vi "Breakdown & Action Taken Report FINAL.vi"(8 "error in (no error)":errorcluster) -> ()   [LabVIEW 2017]
uses:
  <vilib>/Utility/miscctls.llb/LVRowAndColumnTypeDef.ctl
  <vilib>/addons/database/Connection.llb/DB Tools Open Connec (Path).vi
  Globle/Login Details.vi
  <vilib>/Utility/file.llb/Write Delimited Spreadsheet (string).vi
  <vilib>/addons/database/NI_Database_API.lvlib
panel:
  out "Role Id":string
  out "stackholder":string
  in  "Cancel Button - Archive":bool
  out "Table 2":string[][](array[string])
  in  "Manage":bool
  out "Table":string[][](table)
  out "Run-Time Status":cluster{"Array 2":timestamp[], dbl[]}(graph)
  out "index of element":i32
  in  "Download":bool
  in  "Get Rport":bool
  out "subarray":string[](array[string])
  in  "Export to Excel":bool
  in  "Shift":string(combo)
  out "error out":errorcluster
  in  "Station":string(combo)
  in  "To Date":timestamp format="%<%Y-%m-%d>T"
  in  "From Date":timestamp format="%<%Y-%m-%d>T"
  in  "Delete":bool
  in  "Edit":bool
  in  "Select Stakeholder":string(combo)
  in  "Get Report":bool
  # "Breakdown & Action Taken Report"
  # "Designed And Developed By - Infinity Automation Systems Pvt. Ltd."
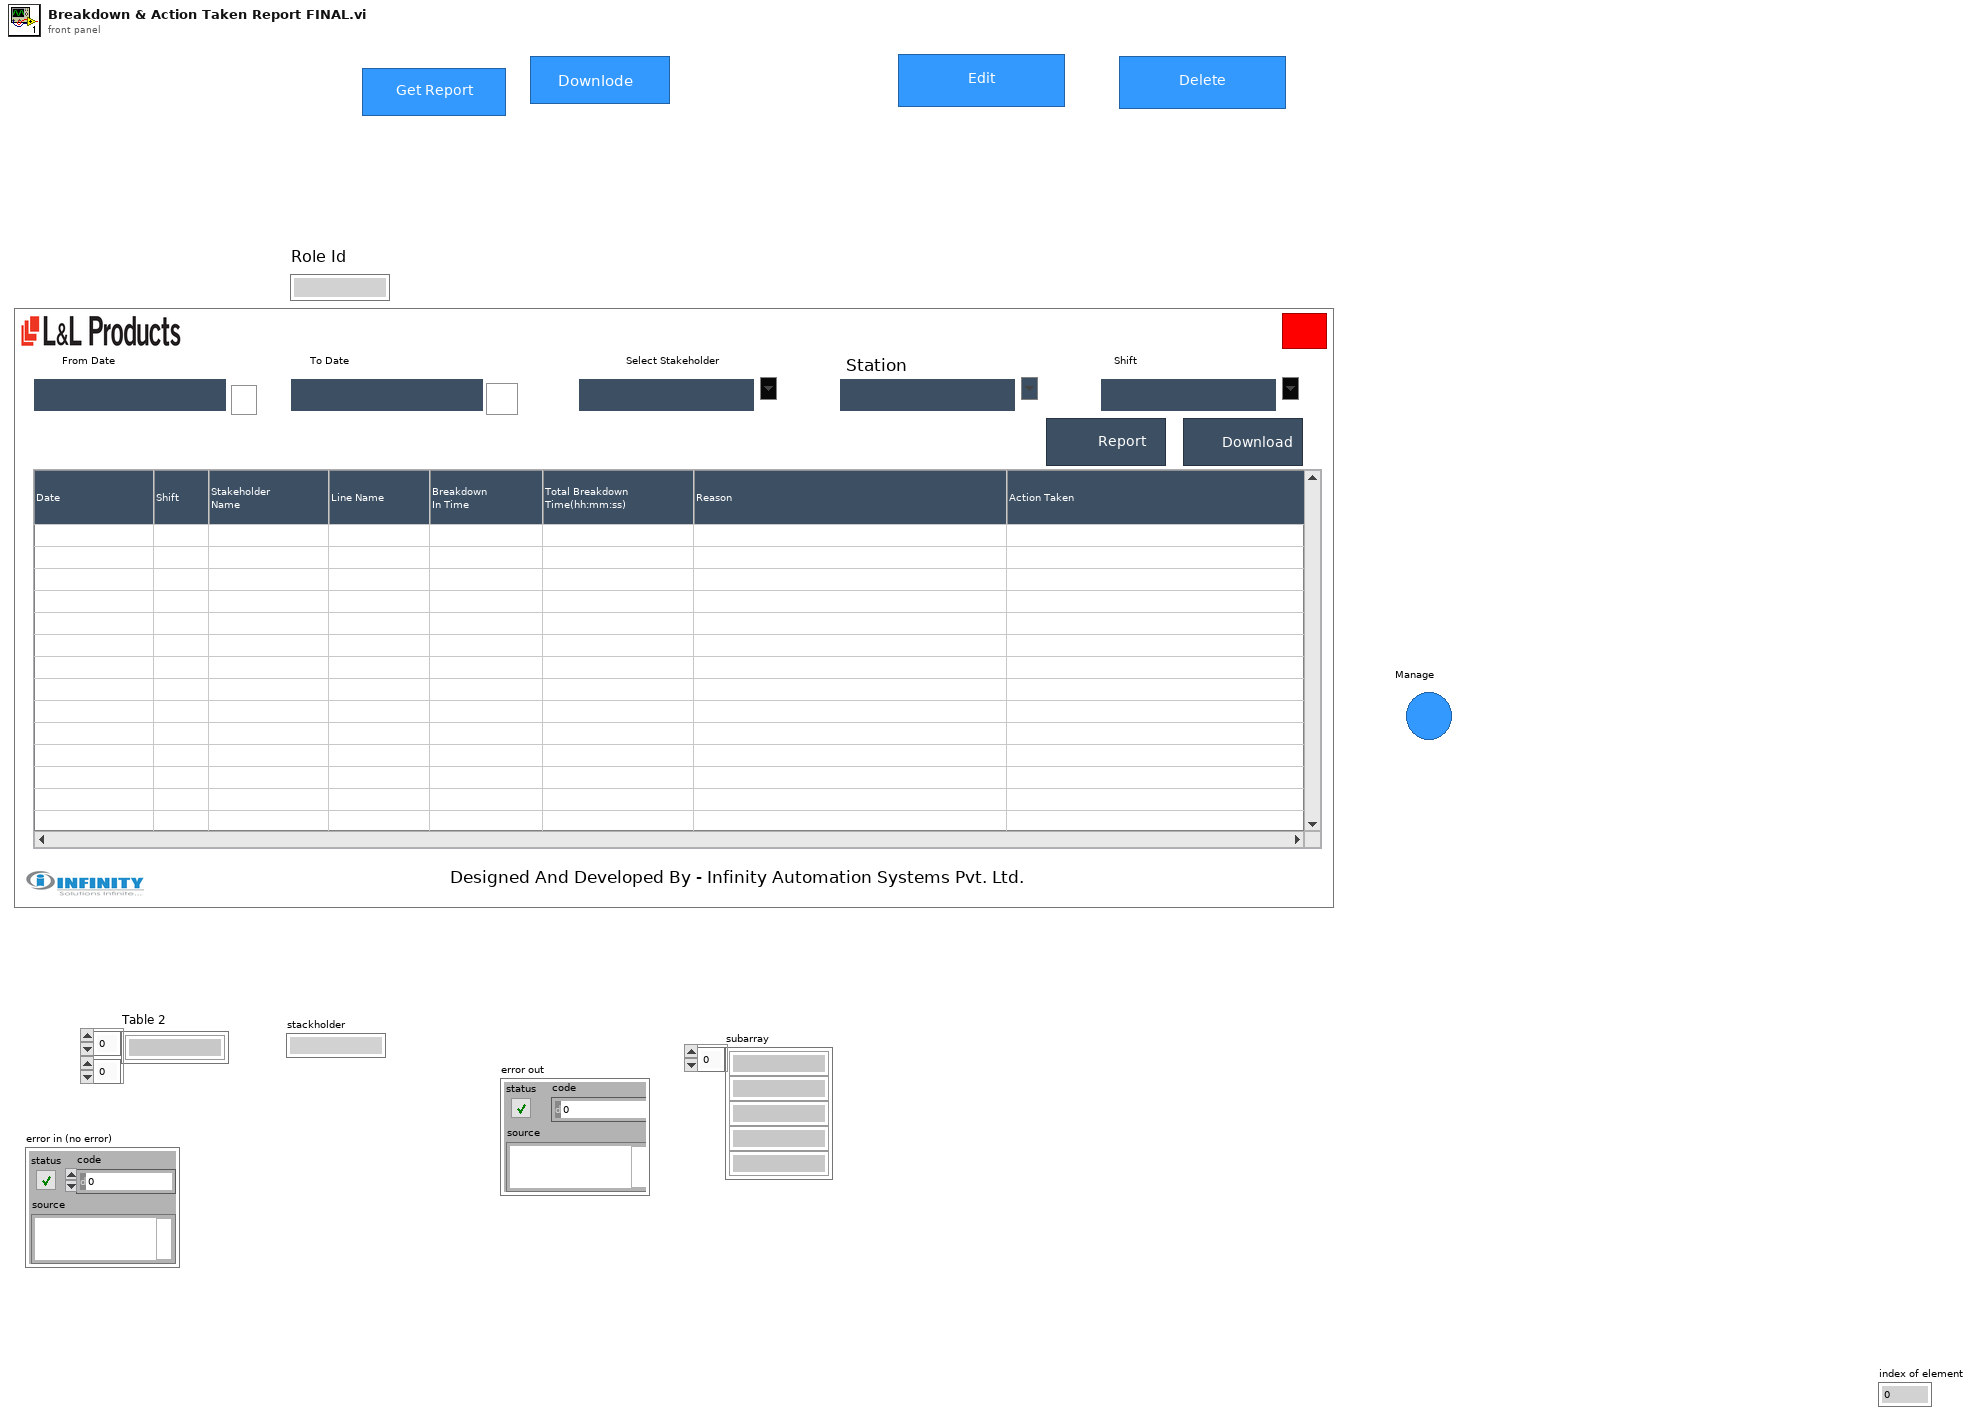
[diagram p1: front panel]
types:
  T1 = typedef "LVRowAndColumnTypeDef.ctl" = cluster{"Row":i32, "Column":i32}
  T2 = typedef "NI_Database_API.lvlib/Conn ObjectReference.ctl" = refnum<k1>
  T3 = enum32{"invalid app kind", "Development System", "Run Time System", "Student Edition", "Embedded LabVIEW", "Evaluation", "Custom"}
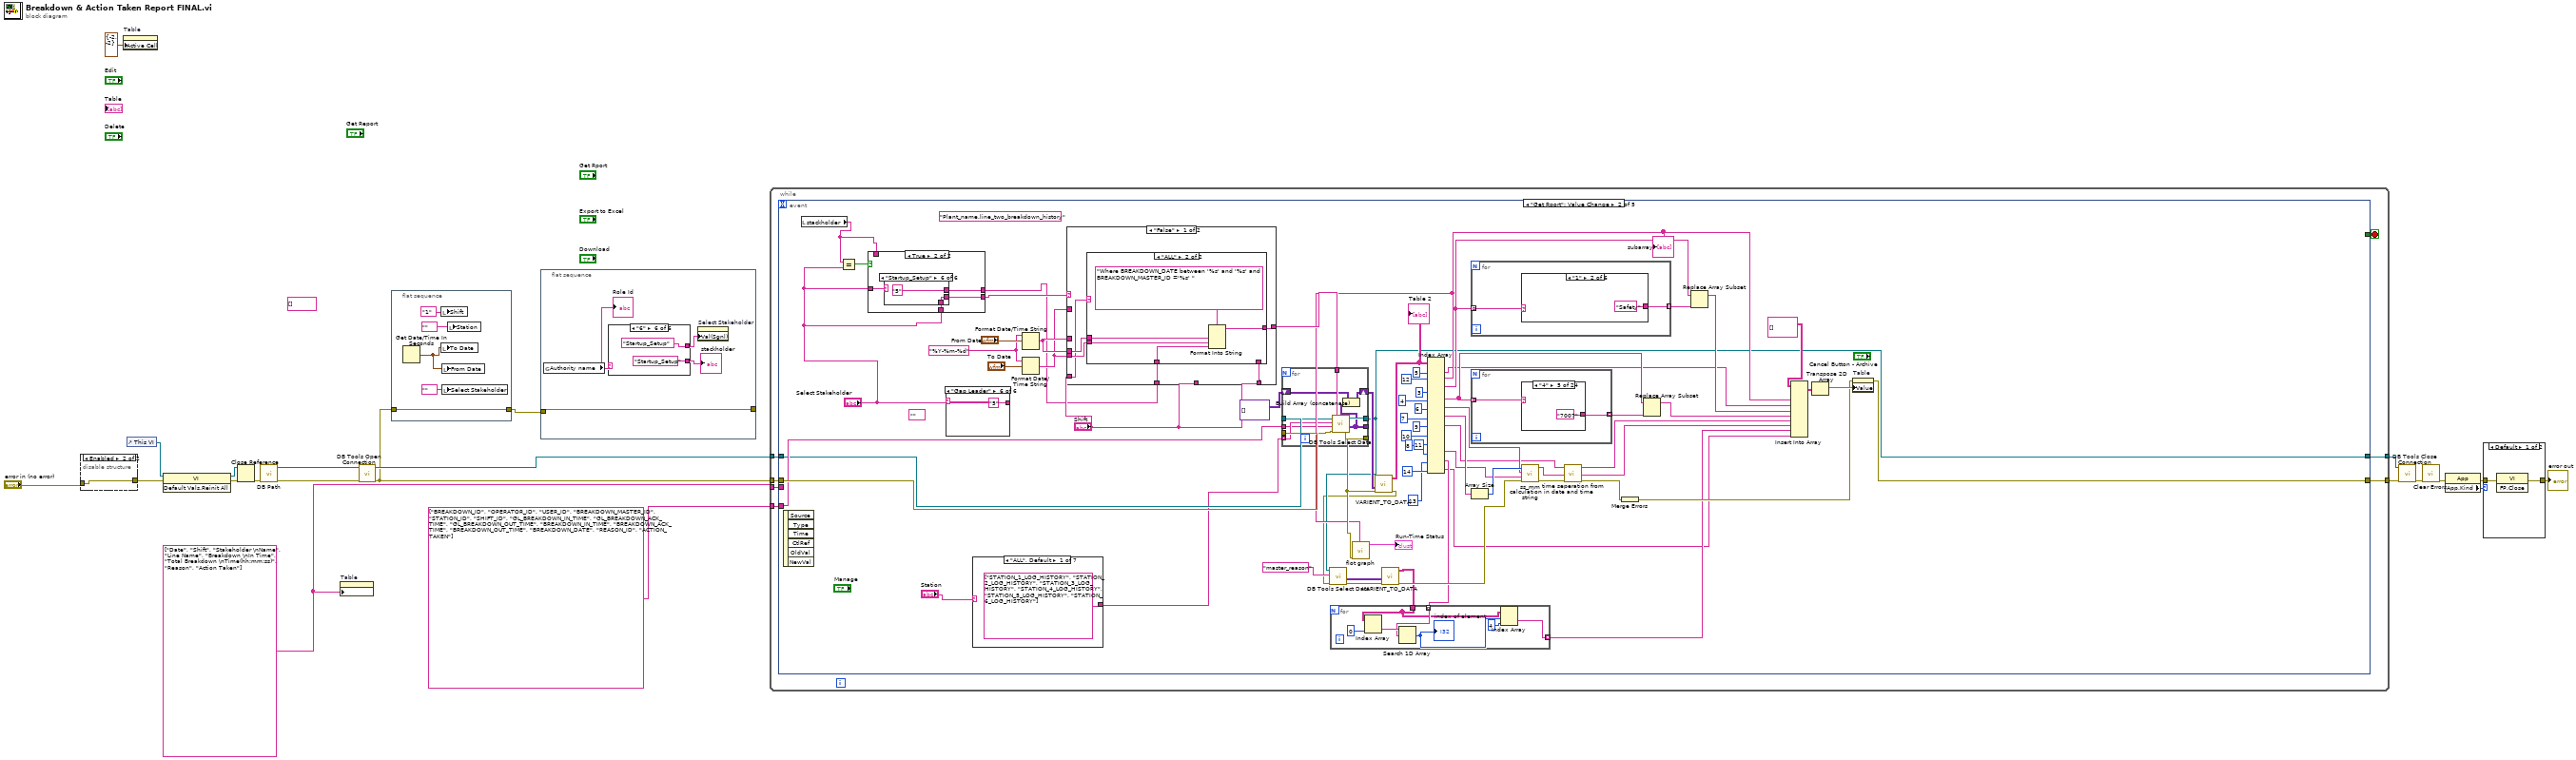
[diagram p0: block diagram]
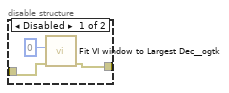
[diagram p2: hidden frame]
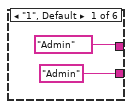
[diagram p3: hidden frame]
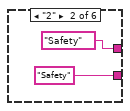
[diagram p4: hidden frame]
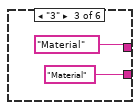
[diagram p5: hidden frame]
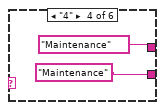
[diagram p6: hidden frame]
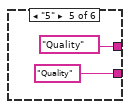
[diagram p7: hidden frame]
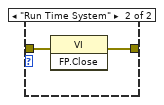
[diagram p8: hidden frame]
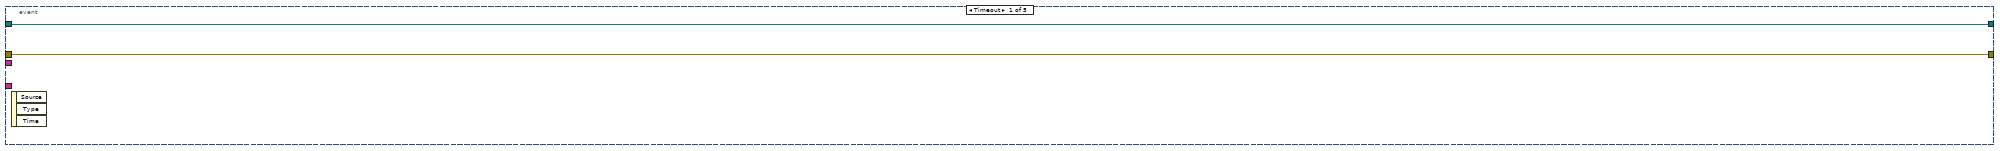
[diagram p9: hidden frame]
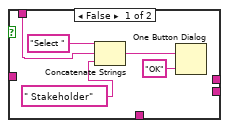
[diagram p10: hidden frame]
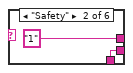
[diagram p12: hidden frame]
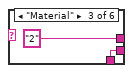
[diagram p13: hidden frame]
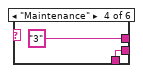
[diagram p14: hidden frame]
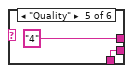
[diagram p15: hidden frame]
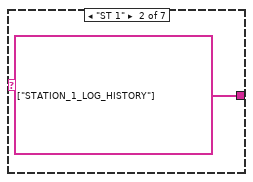
[diagram p16: hidden frame]
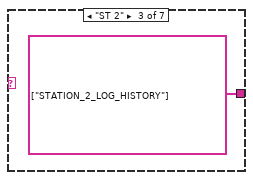
[diagram p17: hidden frame]
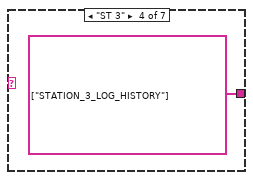
[diagram p18: hidden frame]
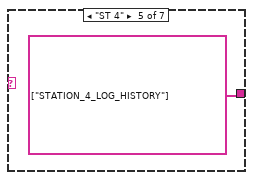
[diagram p19: hidden frame]
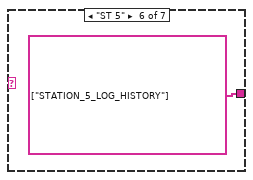
[diagram p20: hidden frame]
diagram:
  (unwired) string[] []
  w5 = string[] ["Date", "Shift", "Stakeholder \nName", "Line Name", "Breakdown \nIn Time", "Total Breakdown \nTime(hh:mm:ss)", "Reason", "Action Taken"] ("Column Header Strings[]")
  n1 = disable-structure shown="Enabled" {
    disable-tunnel: "error in (no error)" -> [w24 w25]
    disable-tunnel: [w23 w25] -> w3
    frame Disabled {
      n2 = call <userlib>:"Fit VI window to Largest Dec__ogtk.vi"("error in (no error)"=w24, "border spacing (2 px)"=0) -> ("error out"=w23:errorcluster)  [unwired: 4 in, 1 out]
    }
    frame Enabled {
    }
  }
  n3 = property on="Table" class="Tbl (strict)"("Active Cell"=T1 {"Row"=-2, "Column"=-2} ("Active Cell:Active Cell")) -> ()  [unwired: 2 in, 2 out]
  n4 = control-ref of="This VI"() -> (w20:refnum<vi>)
  n5 = invoke class="VI" method="Default Vals.Reinit All"(reference=w20, error in=w3) -> (reference out=w18:refnum<vi>, error out=w19:errorcluster)  [unwired: 1 in, 1 out]
  n6 = Close Reference(reference=w18, error in (no error)=w19) -> (error out=w11:errorcluster)
  n7 = call "DB Path.vi"("error in"=w11) -> ("error out"=w10:errorcluster, "DB Path"=w9:path)  [unwired: 9 in]
  n8 = property on="Table" class="Tbl (strict)"("Column Headers[]"=w5) -> ()  [unwired: 2 in, 2 out]
  n9 = call-poly <vilib>:"DB Tools Open Connection.vi"("error in (no error)"=w10, "connection information"=w9) -> ("error out"=w2:errorcluster, "connection reference"=w8:T2)  [unwired: 6 in]
  n10 = flat-sequence {
    tunnel: w2 -> [w26]
    tunnel: [w26] -> w1
    frame #0 {
      n11 = Get Date/Time In Seconds() -> (seconds since 1Jan1904=w30:timestamp)
      n12 = local write "Shift"("1" ("Shift")) -> ()
      n13 = local write "To Date"(w30) -> ()
      n14 = local write "From Date"(w30) -> ()
      n15 = local write "Select Stakeholder"("" ("Select Stakeholder")) -> ()
      n16 = local write "Station"("" ("Select Line")) -> ()
    }
  }
  n17 = flat-sequence {
    tunnel: [w34] -> _
    tunnel: w1 -> [w34]
    frame #0 {
      n18 = global read "Login Details.vi" "Authority name"() -> (w33:string)
      "Role Id" <- w33
      n19 = case shown="\"6\"" w33 {
        tunnel: ["Admin" ("string") "Safety" "Material" "Maintenance" "Quality" "Startup_Setup"] -> w32
        tunnel: ["Admin" ("Stakeholder") "Safety" ("Stakeholder") "Material" ("Stakeholder") "Maintenance" ("Stakeholder") "Quality" ("Stakeholder") "Startup_Setup" ("Stakeholder")] -> w31
        frame "1", Default {
        }
        frame "2" {
        }
        frame "3" {
        }
        frame "4" {
        }
        frame "5" {
        }
        frame "6" {
        }
      }
      "stackholder" <- w32
      n20 = property on="Select Stakeholder" class="CmbBox"("Val(Sgnl)"=w31) -> ()  [unwired: 2 in, 2 out]
    }
  }
  n21 = while {
    tunnel: w2 -> [w53]
    tunnel: [w52] -> w14
    tunnel: [w50] -> w12
    tunnel: w8 -> [w49]
    tunnel: string[] ["BREAKDOWN_ID", "OPERATOR_ID", "USER_ID", "BREAKDOWN_MASTER_ID", "STATION_ID", "SHIFT_ID", "GL_BREAKDOWN_IN_TIME", "GL_BREAKDOWN_ACK_TIME", "GL_BREAKDOWN_OUT_TIME", "BREAKDOWN_IN_TIME", "BREAKDOWN_ACK_TIME", "BREAKDOWN_OUT_TIME", "BREAKDOWN_DATE", "REASON_ID", "ACTION_TAKEN"] ("columns") -> [w48]
    tunnel: w5 -> [w47]
    stop <- w51 stop-if-true
    n22 = event shown="[1] \"Get Rport\": Value Change" {
      selector: _ -> [_ _ _ _ _]
      dyn-events: _ -> [_ _ _ _ _]
      timeout: _ -> [_ _ _ _ _]
      tunnel: w53 -> [w55 w120 w235 w242 _]
      tunnel: [w55 w94 w234 w241 _] -> w52
      tunnel: [_ _ _ _ TRUE] -> w51
      tunnel: [w54 w75 _ _ _] -> w50
      tunnel: w49 -> [w54 w77 _ _ _]
      tunnel: w48 -> [_ w117 _ _ _]
      tunnel: w47 -> [_ _ _ _ _]
      event Timeout {
        n23 = event-data() -> ()  [unwired: 1 in, 3 out]
      }
      event "Get Rport": Value Change {
        (unwired) "" ("Select Stakeholder")
        (unwired) "Plant_name.line_two_breakdown_history" ("table")
        w116 = "%Y-%m-%d" ("time format string (%c)")
        n24 = event-data() -> ()  [unwired: 1 in, 6 out]
        n25 = local read "stackholder"() -> (w59:string)
        n26 = Equal?(x=w59, y="Select Stakeholder") -> (x = y?=w60:bool)
        n27 = case shown="True" w60 {
          tunnel: "Select Stakeholder" -> [_ w129]
          tunnel: w59 -> [w121 _]
          tunnel: "Select Stakeholder" -> [_ w128]
          tunnel: [_ w127] -> w57
          tunnel: [_ w126] -> w56
          frame False {
            n28 = Concatenate Strings("Select " ("message"), w121, " Stakeholder" ("message")) -> (w124:string)
            n29 = One Button Dialog(message=w124, button name ("OK")="OK") -> ()  [unwired: 1 out]
          }
          frame True {
            n30 = case shown="\"Startup_Setup\"" w129 {
              tunnel: w128 -> [w130 w132 w134 w136 w138 w140]
              tunnel: [w130 w132 w134 w136 w138 w140] -> w127
              tunnel: [_ "1" "2" "3" "4" "5"] -> w126
              frame "Admin", Default {
              }
              frame "Safety" {
              }
              frame "Material" {
              }
              frame "Maintenance" {
              }
              frame "Quality" {
              }
              frame "Startup_Setup" {
              }
            }
          }
        }
        n31 = case shown="\"Gap Leader\"" "Select Stakeholder" {
          tunnel: [_ "1" "2" "3" "4" "5"] -> _
          frame "False", Default {
          }
          frame "Logistics" {
          }
          frame "Maintenance" {
          }
          frame "Quality" {
          }
          frame "Production" {
          }
          frame "Gap Leader" {
          }
        }
        n32 = case shown="\"ALL\", Default" "Station" {
          tunnel: [string[] ["STATION_1_LOG_HISTORY", "STATION_2_LOG_HISTORY", "STATION_3_LOG_HISTORY", "STATION_4_LOG_HISTORY", "STATION_5_LOG_HISTORY", "STATION_6_LOG_HISTORY"] string[] ["STATION_1_LOG_HISTORY"] string[] ["STATION_2_LOG_HISTORY"] string[] ["STATION_3_LOG_HISTORY"] string[] ["STATION_4_LOG_HISTORY"] string[] ["STATION_5_LOG_HISTORY"] string[] ["STATION_6_LOG_HISTORY"]] -> w61
          frame "ALL", Default {
          }
          frame "ST 1" {
          }
          frame "ST 2" {
          }
          frame "ST 3" {
          }
          frame "ST 4" {
          }
          frame "ST 5" {
          }
          frame "ST 6" {
          }
        }
        n33 = Format Date/Time String(time format string (%c)=w116, seconds (now)="From Date") -> (date/time string=w91:string)  [unwired: 1 in]
        n34 = Format Date/Time String(time format string (%c)=w116, seconds (now)="To Date") -> (date/time string=w90:string)  [unwired: 1 in]
        n35 = case shown="\"False\"" w57 {
          tunnel: [w165 w182] -> w88
          tunnel: w91 -> [w170 _]
          tunnel: w90 -> [w169 _]
          tunnel: w56 -> [w168 _]
          tunnel: "Shift" -> [w167 w186]
          tunnel: "Shift" -> [w166 _]
          tunnel: w91 -> [_ w185]
          tunnel: w90 -> [_ w184]
          tunnel: "Shift" -> [_ w183]
          frame "False" {
            n36 = case shown="\"ALL\"" w166 {
              tunnel: [w175 w180] -> w165
              tunnel: w170 -> [w174 w179]
              tunnel: w169 -> [w173 w178]
              tunnel: w168 -> [w172 w177]
              tunnel: w167 -> [w171 _]
              frame "False", Default {
                n37 = Format Into String(format string="Where BREAKDOWN_DATE between '%s' and '%s' and BREAKDOWN_MASTER_ID ='%s'  and SHIFT_ID='%s'  " ("condition"), w174, w173, w172, w171) -> (resulting string=w175:string)  [unwired: 2 in, 1 out]
              }
              frame "ALL" {
                n38 = Format Into String(format string="Where BREAKDOWN_DATE between '%s' and '%s' and BREAKDOWN_MASTER_ID ='%s' " ("condition"), w179, w178, w177) -> (resulting string=w180:string)  [unwired: 2 in, 1 out]
              }
            }
          }
          frame "Admin", Default {
            n39 = case shown="\"ALL\"" w186 {
              tunnel: w185 -> [w190 w194]
              tunnel: w184 -> [w189 w193]
              tunnel: w183 -> [w188 _]
              tunnel: [w187 w192] -> w182
              frame "False", Default {
                n40 = Format Into String(format string="Where BREAKDOWN_DATE between '%s' and '%s' and SHIFT_ID='%s'  " ("condition"), w190, w189, w188) -> (resulting string=w187:string)  [unwired: 2 in, 1 out]
              }
              frame "ALL" {
                n41 = Format Into String(format string="Where BREAKDOWN_DATE between '%s' and '%s'" ("condition"), w194, w193) -> (resulting string=w192:string)  [unwired: 2 in, 1 out]
              }
            }
          }
        }
        n42 = for {
          tunnel: w61 -> [w162] mode=indexing
          tunnel: [w156] -> _
          tunnel: w117 -> [w158]
          tunnel: w88 -> [w159]
          tunnel: w120 -> [w161]
          tunnel: [w160] -> w93
          tunnel: w77 -> [w164]
          tunnel: [w163] -> w75
          shift-right: [w155] -> w86
          shift-left: variant[][] [] ("data") -> [w157]
          n43 = call <vilib>:"DB Tools Select Data.vi"("condition"=w159, "error in (no error)"=w161, "columns"=w158, "table"=w162, "connection reference"=w164) -> ("error out"=w160:errorcluster, "data"=w156:variant[][], "connection reference out"=w163:T2)  [unwired: 1 in]
          n44 = Build Array (concatenate)(w157, w156) -> (w155:variant[][])
        }
        n45 = call "VARIENT_TO_DATA.vi"("data"=w86, "error in (no error)"=w93) -> ("Table"=w80:string[][], "error out"=w73:errorcluster)  [unwired: 7 in]
        "Table 2" <- w80
        n46 = call <vilib>:"DB Tools Select Data.vi"("error in (no error)"=w73, "table"="master_reason", "connection reference"=w75) -> ("error out"=w76:errorcluster, "data"=w74:variant[][])  [unwired: 3 in, 1 out]
        n47 = call "VARIENT_TO_DATA.vi"("data"=w74, "error in (no error)"=w76) -> ("Table"=w71:string[][], "error out"=w72:errorcluster)  [unwired: 7 in]
        n48 = Index Array(array=w80, index (col) #1=5 ("disabled index (col)"), index (col) #2=12 ("disabled index (col)"), index (col) #3=3 ("index (col)"), index (col) #4=4 ("index (col)"), index (col) #5=6 ("index (col)"), index (col) #6=7 ("index (col)"), index (col) #7=9 ("index (col)"), index (col) #8=10 ("index (col)"), index (col) #9=11 ("index (col)"), index (col) #10=8 ("index (col)"), index (col) #11=13 ("index (col)"), index (col) #12=14 ("index (col)")) -> (element #1=w82:string[], element #2=w83:string[], element #3=w113:string[], element #4=w100:string[], element #5=w68:string[], element #6=w97:string[], element #7=w63:string[], element #10=w95:string[], element #11=w70:string[], element #12=w64:string[])  [unwired: 12 in, 2 out]
        "subarray" <- w83
        n49 = for {
          tunnel: w71 -> [w148]
          tunnel: w70 -> [w150] mode=indexing
          tunnel: [w149] -> w65 mode=indexing
          n50 = Index Array(array=w148, index (col)=0 ("disabled index (col)")) -> (element=w153:string[])  [unwired: 1 in]
          n51 = Search 1D Array(1D array=w153, element=w150) -> (index of element=w154:i32)  [unwired: 1 in]
          "index of element" <- w154
          n52 = Index Array(array=w148, index (row)=w154, index (col)=4 ("disabled index (col)")) -> (element=w149:string)
        }
        n53 = call "flot graph.vi"("BD Date"=w83, "error in (no error)"=w93) -> ("Run-Time Status"=→"Run-Time Status":cluster{"Array 2":timestamp[], dbl[]})  [unwired: 9 in]
        n54 = for {
          tunnel: w113 -> [w222] mode=indexing
          tunnel: [w221] -> w112 mode=indexing
          n55 = case shown="\"1\"" w222 {
            tunnel: ["all" "Safety" "Material" "Maintenance" "Quality" "Startup_Setup"] -> w221
            frame "False", Default {
            }
            frame "1" {
            }
            frame "2" {
            }
            frame "3" {
            }
            frame "4" {
            }
            frame "5" {
            }
          }
        }
        n56 = for {
          tunnel: w100 -> [w197] mode=indexing
          tunnel: [w196] -> w99 mode=indexing
          n57 = case shown="\"4\"" w197 {
            tunnel: [_ "7001" "7002" "7004" "7007" "7006" "7008" "HVI" "7009" "SA" "M&M" "TML" "5001" "1001" "4003" "1002" "4004" "1004" "2001" "3001" "2004" "3002" "3003" "4001"] -> w196
            frame "0", Default {
            }
            frame "1" {
            }
            frame "2" {
            }
            frame "3" {
            }
            frame "4" {
            }
            frame "5" {
            }
            frame "6" {
            }
            frame "7" {
            }
            frame "8" {
            }
            frame "9" {
            }
            frame "10" {
            }
            frame "11" {
            }
            frame "12" {
            }
            frame "13" {
            }
            frame "14" {
            }
            frame "15" {
            }
            frame "16" {
            }
            frame "17" {
            }
            frame "18" {
            }
            frame "19" {
            }
            frame "20" {
            }
            frame "21" {
            }
            frame "22" {
            }
            frame "23" {
            }
          }
        }
        n58 = Array Size(array=w97) -> (size(s)=w96:i32)
        n59 = call "ss_mm calculation in string.vi"("error in (no error)"=w72, "Table 2"=w95, "Table"=w68, "Numeric"=w96) -> ("error out"=w85:errorcluster, "Array 2"=w66:string[])  [unwired: 6 in]
        n60 = call "time seperation from  date and time.vi"("time and date"=w63) -> ("time array"=w67:string[])  [unwired: 10 in]
        n61 = Merge Errors(w85) -> (w69:errorcluster)
        n62 = Replace Array Subset(array=w100, new element=w99) -> (w98:string[])  [unwired: 1 in]
        n63 = Replace Array Subset(array=w113, new element=w112) -> (w110:string[])  [unwired: 1 in]
        n64 = Insert Into Array(array=string[][] [], new element #1=w83, new element #2=w82, new element #3=w110, new element #4=w98, new element #5=w67, new element #6=w66, new element #7=w65, new element #8=w64) -> (w109:string[][])  [unwired: 2 in]
        n65 = Transpose 2D Array(2D array=w109) -> (transposed array=w108:string[][])
        n66 = property on="Table" class="Tbl (strict)"(error in=w69, "Value"=w108) -> (error out=w94:errorcluster)  [unwired: 1 in, 1 out]
      }
      event "Manage": Value Change {
        n67 = event-data() -> ()  [unwired: 1 in, 6 out]
        n68 = disable-structure shown="Disabled" {
          disable-tunnel: w235 -> [w237 _]
          disable-tunnel: [w236 _] -> w234
          frame Disabled {
            n69 = call "manage breakdown sub.vi"("error in (no error)"=w237) -> ("error out"=w236:errorcluster)  [unwired: 10 in]
          }
          frame Enabled {
          }
        }
      }
      event "Download": Value Change {
        n70 = event-data() -> ()  [unwired: 1 in, 6 out]
        n71 = call "File Dialog"() -> ("selected path"=w246:path, "error out"=w245:errorcluster)  [unwired: 12 in, 2 out]
        n72 = call <vilib>:"Clear Errors.vi"("error in (no error)"=w245) -> ()  [unwired: 5 in, 2 out]
        n73 = Path To String(path=w246) -> (string=w247:string)
        n74 = Concatenate Strings(w247, ".csv" ("string")) -> (w248:string)
        n75 = property on="Table" class="Tbl (strict)"() -> ("Value"=w243:string[][])  [unwired: 2 in, 2 out]
        n76 = String To Path(string=w248) -> (path=w249:path)
        n77 = Build Array (concatenate)(string[][] [["Date", "Stakeholder Name", "Line Name", "Breakdown In Time", "Total Breakdown Time(mm.ss)", "Reason", "Action Taken"]] ("Column Header Strings[]"), w243) -> (w238:string[][])
        n78 = call-poly <vilib>:"Write Delimited Spreadsheet.vi"("file path (dialog if empty)"=w249, "2D data"=w238, "error in (no error)"=w242, "delimiter (\\t)"="," ("delimiter (\\t)")) -> ("error out"=w241:errorcluster)  [unwired: 10 in, 1 out]
      }
      event "Cancel Button - Archive": Value Change {
        n79 = event-data() -> ()  [unwired: 1 in, 6 out]
      }
    }
  }
  n80 = call <vilib>:"DB Tools Close Connection.vi"("error in (no error)"=w14, "connection reference"=w12) -> ("error out"=w15:errorcluster)  [unwired: 5 in]
  n81 = call <vilib>:"Clear Errors.vi"("error in (no error)"=w15) -> ("error out"=w13:errorcluster)  [unwired: 5 in, 1 out]
  n82 = property class="App"(error in=w13) -> (error out=w16:errorcluster, "App.Kind"=w17:T3)  [unwired: 1 in, 1 out]
  n83 = case shown="Default" w17 {
    tunnel: w16 -> [w252 w254]
    tunnel: [w251 w253] -> w6
    frame Default {
      n84 = invoke class="VI" method="FP.Close"(error in=w252) -> (error out=w251:errorcluster)  [unwired: 2 in, 2 out]
    }
    frame "Run Time System" {
      n85 = invoke class="VI" method="FP.Close"(error in=w254) -> (error out=w253:errorcluster)  [unwired: 2 in, 2 out]
    }
  }
  "error out" <- w6
